vi "Set and Get ItemNames With Symbol.vi"(7 "Mode":T3, 8 "错误输入":errorcluster, 10 "ItemNames In":T1[](array[typedef]), 11 "Listbox Ref":refnum<vi>) -> (0 "错误输出":errorcluster, 2 "ItemNames Out":T1[](array[typedef]), 3 "Dup Listbox Ref":refnum<vi>)   [LabVIEW 2012, in "Listbox Tool.lvlib"]
uses:
  Listbox Tool.lvlib
  Custom Type/Read and Write Mode.ctl
  ItemName With Symbol.ctl
  Custom Type/System Symbols.ctl
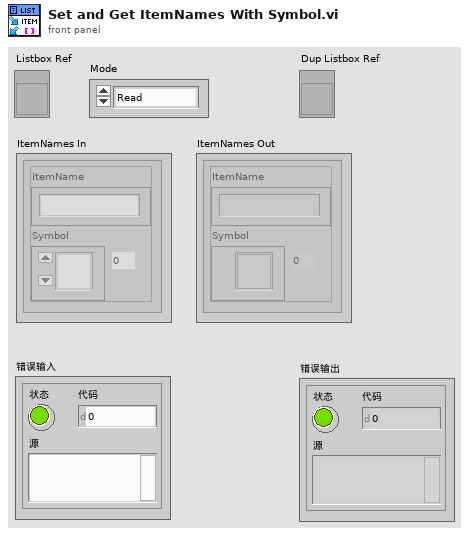
[diagram p1: front panel]
types:
  T1 = typedef "Listbox Tool.lvlib/ItemName With Symbol.ctl" = cluster{"ItemName":string, "Symbol":T2}
  T2 = typedef "Listbox Tool.lvlib/System Symbols.ctl" = i32
  T3 = typedef "Listbox Tool.lvlib/Read and Write Mode.ctl" = enum16{"Read", "Write"}
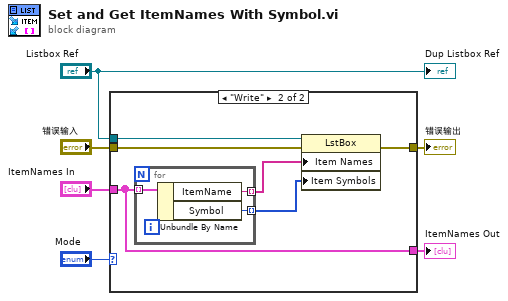
[diagram p0: block diagram]
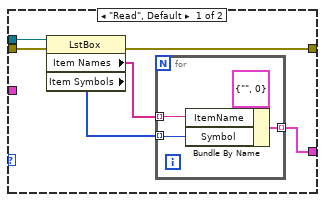
[diagram p2: hidden frame]
diagram:
  n1 = case shown="\"Write\"" "Mode" {
    tunnel: "Listbox Ref" -> [w11 w22]
    tunnel: "错误输入" -> [w12 w21]
    tunnel: [w10 w20] -> w4
    tunnel: [w7 w17] -> w2
    tunnel: "ItemNames In" -> [_ w17]
    frame "Read", Default {
      n2 = property class="LstBox"(reference=w11, error in=w12) -> (error out=w10:errorcluster, "Item Names"=w9:string[], "Item Symbols"=w8:i32[])  [unwired: 1 out]
      n3 = for {
        tunnel: w9 -> [w15] mode=indexing
        tunnel: w8 -> [w14] mode=indexing
        tunnel: [w13] -> w7 mode=indexing
        n4 = Bundle By Name(cluster=T1 {"ItemName"="", "Symbol"=0} ("Name With Symbol"), "ItemName"=w15, "Symbol"=w14) -> (w13:T1)
      }
    }
    frame "Write" {
      n5 = for {
        tunnel: w17 -> [w25] mode=indexing
        tunnel: [w24] -> w19 mode=indexing
        tunnel: [w23] -> w18 mode=indexing
        n6 = Unbundle By Name(w25) -> ("ItemName"=w24:string, "Symbol"=w23:T2)
      }
      n7 = property class="LstBox"(reference=w22, error in=w21, "Item Names"=w19, "Item Symbols"=w18) -> (error out=w20:errorcluster)  [unwired: 1 out]
    }
  }
  "错误输出" <- w4
  "ItemNames Out" <- w2
  "Dup Listbox Ref" <- "Listbox Ref"
